vi "Pivot power increase.vi"(7 "Pivot Increase":dbl min=0.0 max=0.5 step=0.1, 9 "Input Pivot Right":dbl, 11 "Input Pivot Left":dbl) -> (1 "Output Pivot Right":dbl, 3 "Output Pivot Left":dbl)   [LabVIEW 2019]
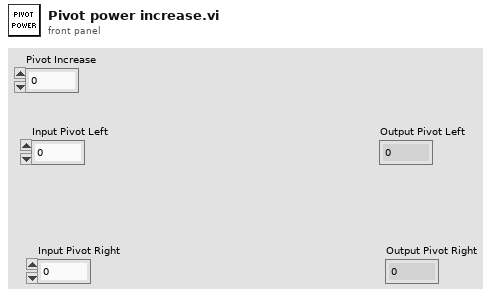
[diagram p1: front panel]
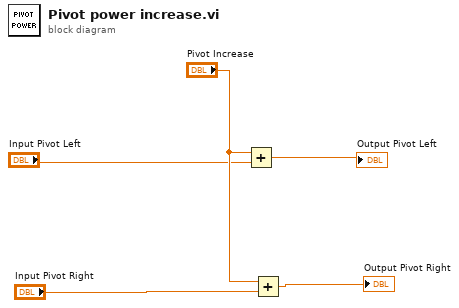
[diagram p0: block diagram]
diagram:
  n1 = Add(x="Pivot Increase", y="Input Pivot Left") -> (x+y=→"Output Pivot Left":dbl)
  n2 = Add(x="Pivot Increase", y="Input Pivot Right") -> (x+y=→"Output Pivot Right":dbl)
